vi "曲线.vi"() -> ()   [LabVIEW 2020]
panel:
  out "Tab Control":enum32{"力特性", "内泄露", "压销位移力曲线"}(tab)
  out "力特性":cluster{dbl[], dbl[]}[](graph)
  out "内泄露":cluster{dbl[], dbl[]}[](graph)
  out "压力位移曲线":cluster{dbl[], dbl[]}[](graph)
  in  "停止":bool
  # "力特性试验"
  # "内泄露试验"
  # "压销位移力曲线"
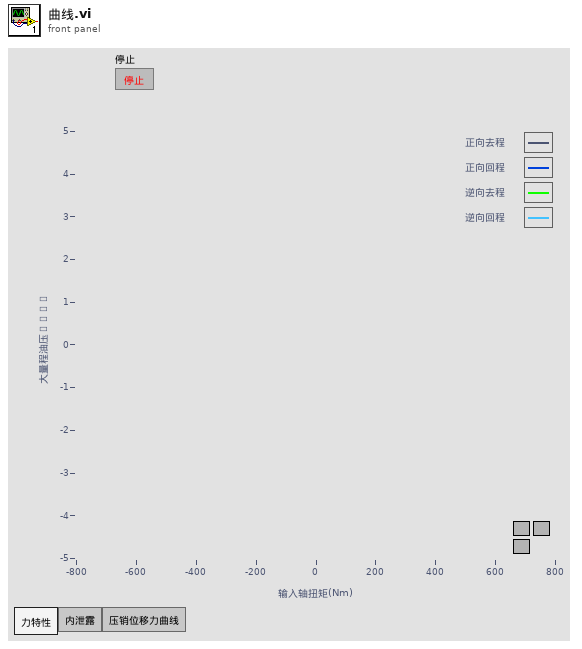
[diagram p1: front panel]
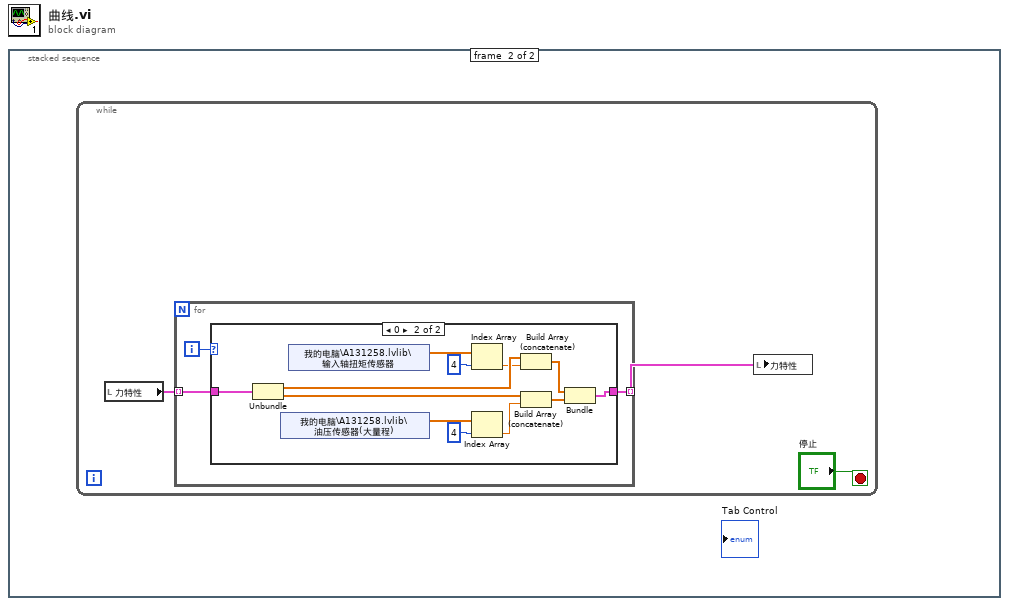
[diagram p0: block diagram]
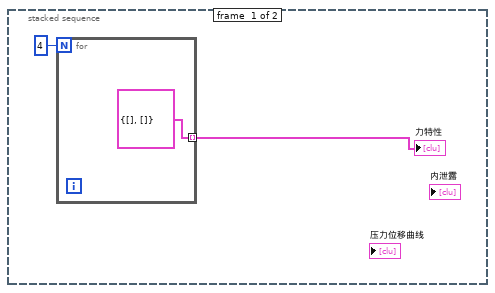
[diagram p2: hidden frame]
diagram:
  n1 = stacked-sequence {
    frame #0 {
      n2 = for {
        N: 4 -> [_]
        tunnel: [cluster{dbl[], dbl[]} {[], []}] -> w1 mode=indexing
      }
      "力特性" <- w1
    }
    frame #1 {
      n3 = while {
        stop <- "停止" stop-if-true
        n4 = local read "力特性"() -> (w5:cluster{dbl[], dbl[]}[])
        n5 = for {
          tunnel: [w9] -> w6 mode=indexing
          tunnel: w5 -> [w8] mode=indexing
          i -> [w7]
          n6 = case shown="0" w7 {
            tunnel: [w10 w14] -> w9
            tunnel: w8 -> [w10 w13]
            frame Default {
            }
            frame 0 {
              n7 = Unbundle(w13) -> (w18:dbl[], w17:dbl[])
              n8 = shared-variable "我的电脑\\A131258.lvlib\\油压传感器(大量程)"() -> (w22:sgl[])  [unwired: 1 in, 1 out]
              n9 = shared-variable "我的电脑\\A131258.lvlib\\输入轴扭矩传感器"() -> (w20:sgl[])  [unwired: 1 in, 1 out]
              n10 = Index Array(array=w20, index=4) -> (element=w11:sgl)
              n11 = Index Array(array=w22, index=4) -> (element=w12:sgl)
              n12 = Build Array (concatenate)(w18, w11) -> (w16:dbl[])
              n13 = Build Array (concatenate)(w17, w12) -> (w15:dbl[])
              n14 = Bundle(w16, w15) -> (w14:cluster{dbl[], dbl[]})  [unwired: 1 in]
            }
          }
        }
        n15 = local write "力特性"(w6) -> ()
      }
    }
  }
